vi "main_control_combo.vi"(6 "read":bool=TRUE) -> (9 "read string":string, 10 "bytes read":u32)   [LabVIEW 2019]
doc: "The Basic Serial Read and Write example performs a Serial Port Read, a Serial Port Write, or a combination of these actions. The user selects the actions (read or write) on the front panel. If both are selected, the VI will write the data first, read data, and then close the VISA session that is opened to the port. This VI will wait until the specified number of bytes is received at the port. Only the number of bytes specified will be read.\n\nINSTRUCTIONS:\n1) Select the serial resource and configuration parameters (baud rate, data bits, parity, stop bits, flow control).\n2) Select the operations to be performed. \n3) Connect the serial port to your device. If no device is available, perform a loopback test by doing one of the following. Short pins 2 and 3 on a RS-232 cable or short pin 4 to pin 8 and pin 5 to pin 9 on a RS-485/422 cable. \n4) Run the VI to see the data read. (The \"read string\" will match the \"string to write\" if a loopback test was performed.)\n\nNote: The parameters set for the serial port must match the parameters of the connected instrument or device. In this example, the bytes to read parameter specifies the number of bytes that the serial port reads. If there were more bytes at the port than the number specified in bytes to read, those bytes would not be read. Also, if you specify to read more bytes than the number of bytes actually read, you might receive a timeout error message.\n\nOn the block diagram, the Configure Serial Port VI sets the configuration parameters. The front panel displays the controls used to configure the basic parameters, such as baud rate, data bits, and parity. Constants configure the other parameters the user probably does not need set. After the VISA Configure Serial Port VI opens the VISA session and configures the port, the VI passes the VISA resource name to other VIs that perform operations on that VISA resource. The VISA Write function sends a command to the serial device and the VISA Read function returns data based on the command. The VISA Close function then closes the reference to the serial device. It is important to close the reference; otherwise communication through with that port through protocols other than VISA might not be possible."
uses:
  <vilib>/Instr/_visa.llb/VISA Configure Serial Port (Instr).vi
  <vilib>/Utility/file.llb/Read Delimited Spreadsheet (string).vi
  Keithley/Keithley 24XX/Public/Data/Read (Single Point).vi
  Keithley/Keithley 24XX/Keithley 24XX.lvlib
  DELTA ELEKTRONIKA SM Series/DELTA ELEKTRONIKA.lvlib
panel:
  out "Current Limit 2":bool
  out "Voltage Limit 2":bool
  out "bytes read 5":u32
  out "read string 5":string
  out "bytes read 4":u32
  out "read string 4":string
  out "standard output":string
  in  "Voltage Manual Range (1.0) 2":dbl=1.0
  in  "Current Manual Range (1.0) 2":dbl=1.0
  in  "Resistance Manual Range (1.0) 2":dbl=1.0
  in  "Enable Voltage Auto Range (T:Enable) 2":bool=TRUE
  in  "Enable Current Auto Range (T:Enable) 2":bool=TRUE
  in  "Enable Resistance Auto Range (T:Enable) 2":bool=TRUE
  out "Voltage 3":sgl
  out "Current 3":sgl
  out "Resistance 2":sgl
  out "Current Micro\n 2":sgl
  out "Command Log and Output":string
  out "COMBO COMMAND":string
  in  "Current Limit (0A)":dbl format="%.2f"
  in  "Voltage Level (0.0 V)":dbl format="%.2f"
  out "Actual Voltage Level (V)":dbl format="%.2f"
  out "Actual Current Limit (A)":dbl format="%.2f"
  out "Voltage Limit":bool
  out "Current Limit":bool
  out "all rows":string[][](array[string])
  out "element":i32
  out "subarray 4":string[](array[string])
  out "subarray 5":string[](array[string])
  out "size(s)":i32
  in  "file path (dialog if empty) 2":path
  in  "Read Script":bool
  in  "Voltage Manual Range (1.0)":dbl=1.0
  in  "Current Manual Range (1.0)":dbl=1.0
  in  "Resistance Manual Range (1.0)":dbl=1.0
  in  "Enable Voltage Auto Range (T:Enable)":bool=TRUE
  in  "Enable Current Auto Range (T:Enable)":bool=TRUE
  in  "Enable Resistance Auto Range (T:Enable)":bool=TRUE
  out "relay TTi":errorcluster
  out "bytes read 3":u32
  out "read string 3":string
  in  "read 3":bool=TRUE
  in  "delay before read (ms) 3":u32=500
  in  "Combo Box 3":string(combo)
  in  "voltage or current 2":dbl
  out "string from combo 3":string
  in  "write 3":bool
  out "LV TTi":errorcluster
  out "bytes read 2":u32
  out "read string 2":string
  in  "read 2":bool=TRUE
  in  "delay before read (ms) 2":u32=500
  in  "Combo Box 2":string(combo)="VO?\n"
  in  "voltage or current":dbl
  out "string from combo 2":string
  in  "write 2":bool
  in  "write":bool
  out "string from combo":string
  in  "Temperature":dbl
  in  "Combo Box":string(combo)
  out "Chiller":errorcluster
  out "N2 temperature > dew point + 2C":bool
  in  "File Path of rotonic datalog":path
  out "time humidity temporature dewpoint":string[](array[string])
  in  "Quit":bool
  in  "delay before read (ms)":u32=500
  # "Medical Chiller Interface\nCOM 6 is default"
  # "TTi LV powersupply Interface\nCOM 5 is default"
  # "TTi LV powersupply Interface for the relay polarity control\nCOM 4 is default"
  # "µA"
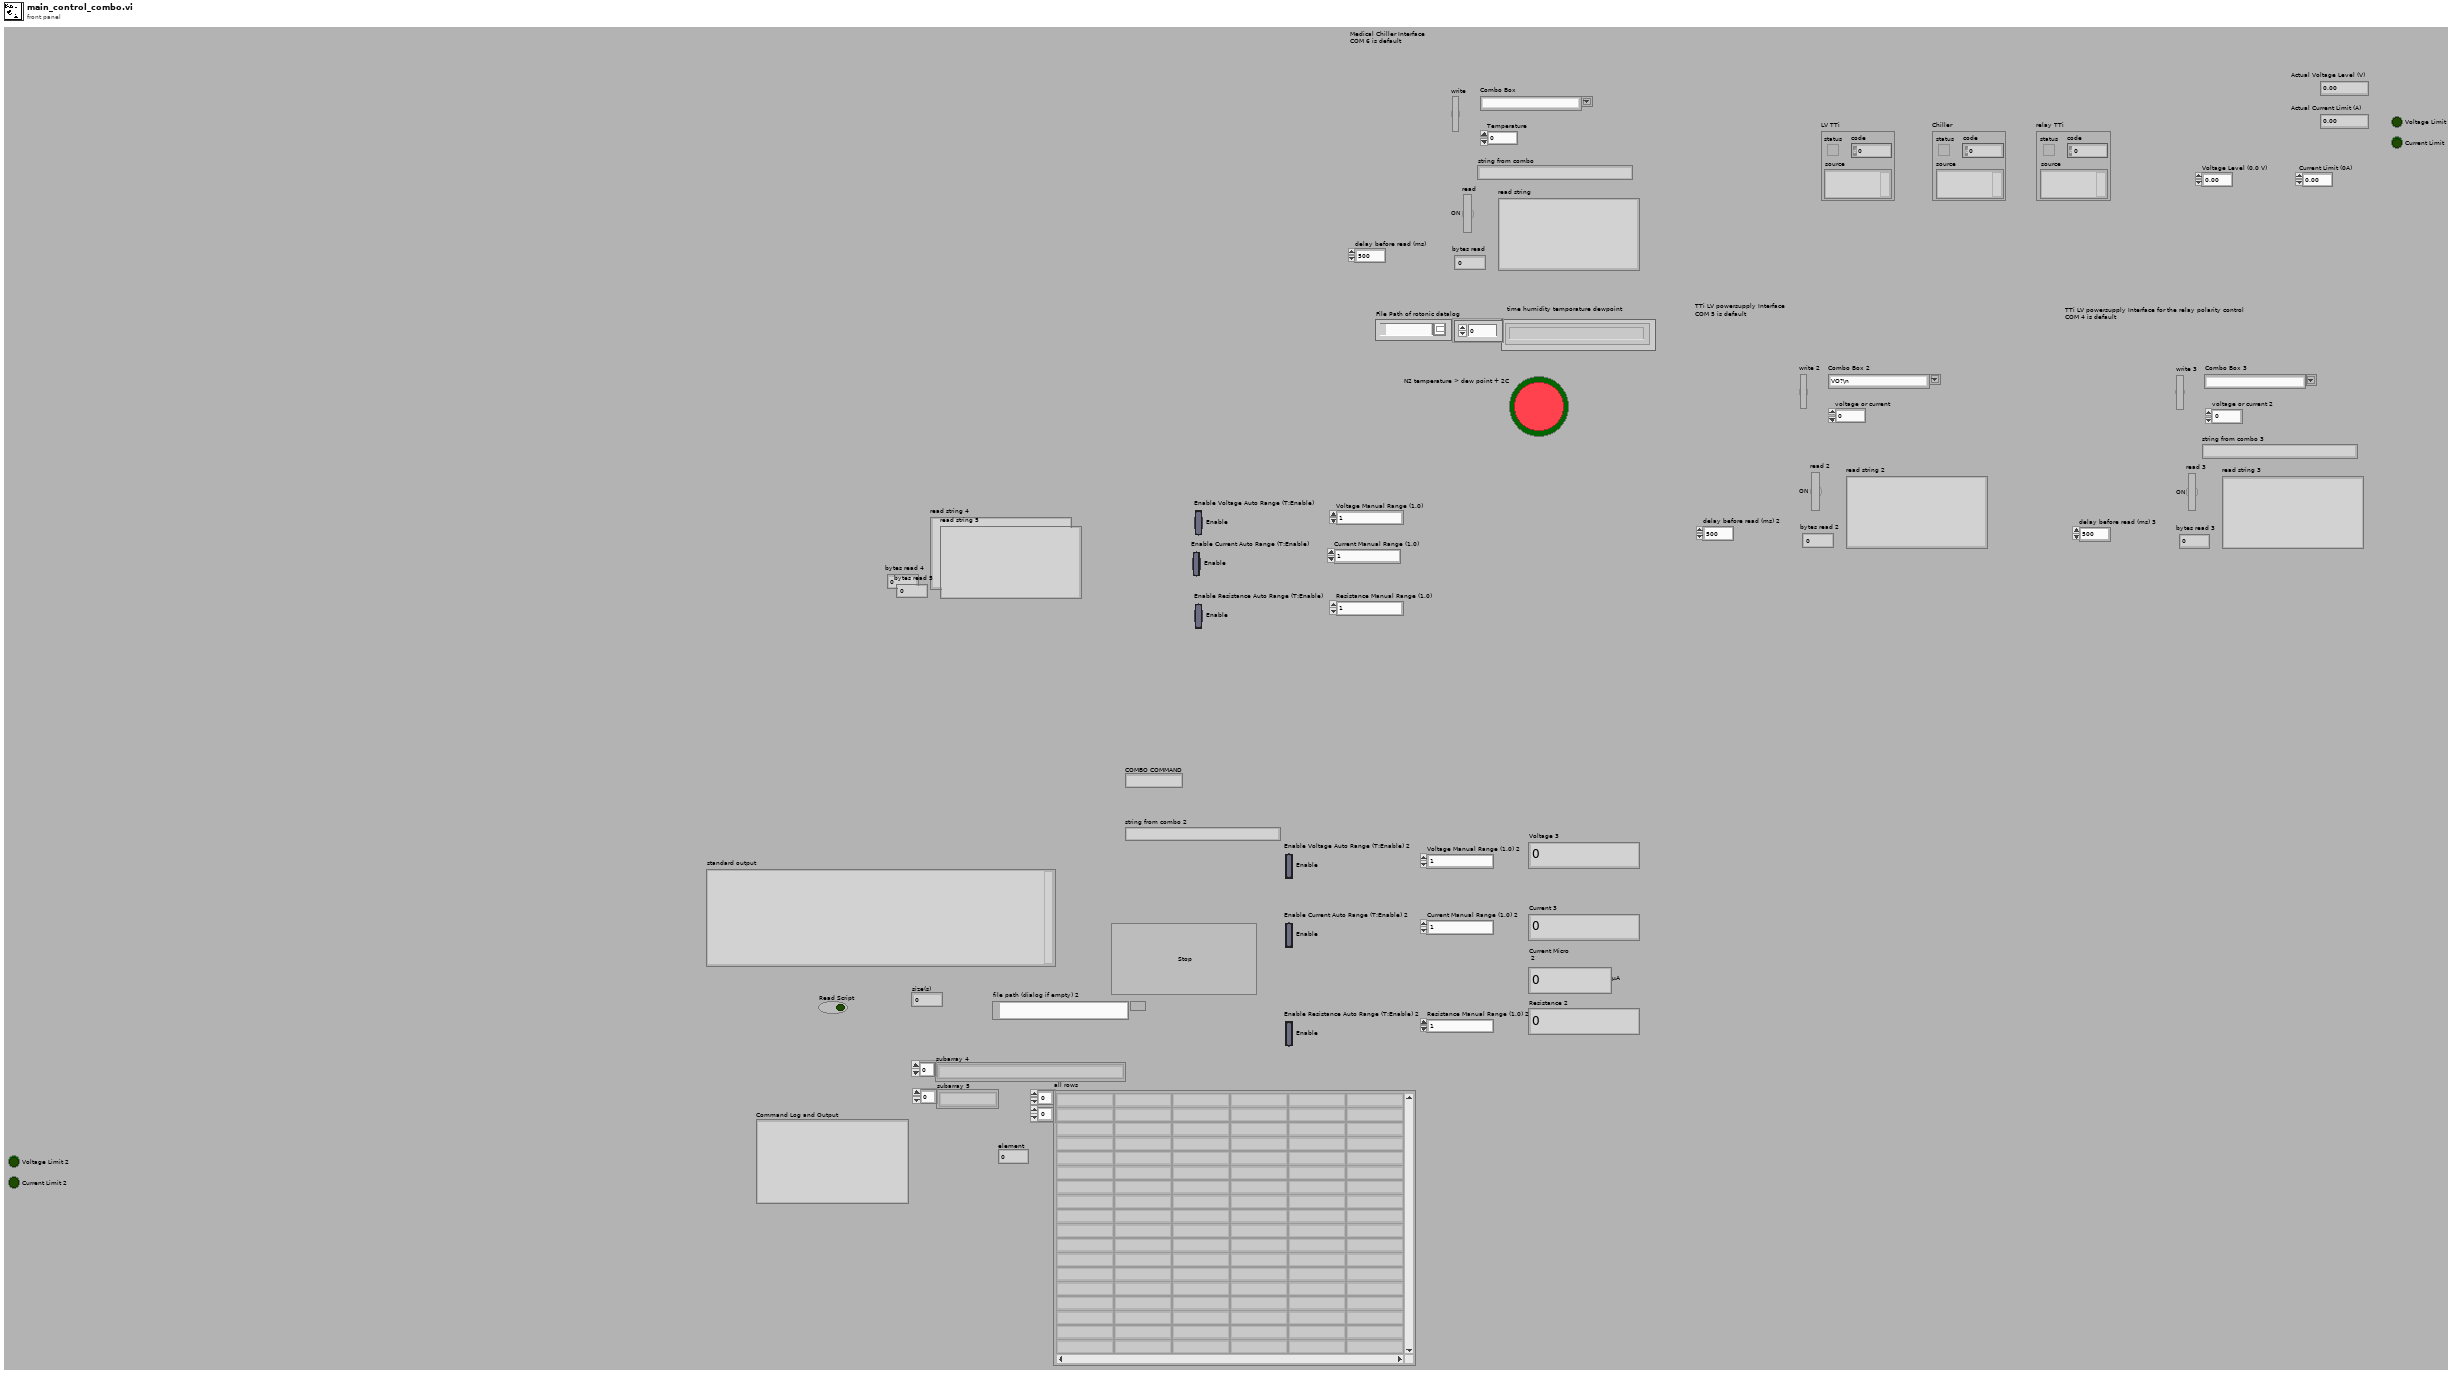
[diagram p1: front panel]
types:
  T1 = cluster{"Baud Rate":u32, "Parity":u16, "Data Bits":u16, "Stop Bits":u16, "Flow Control":u16}
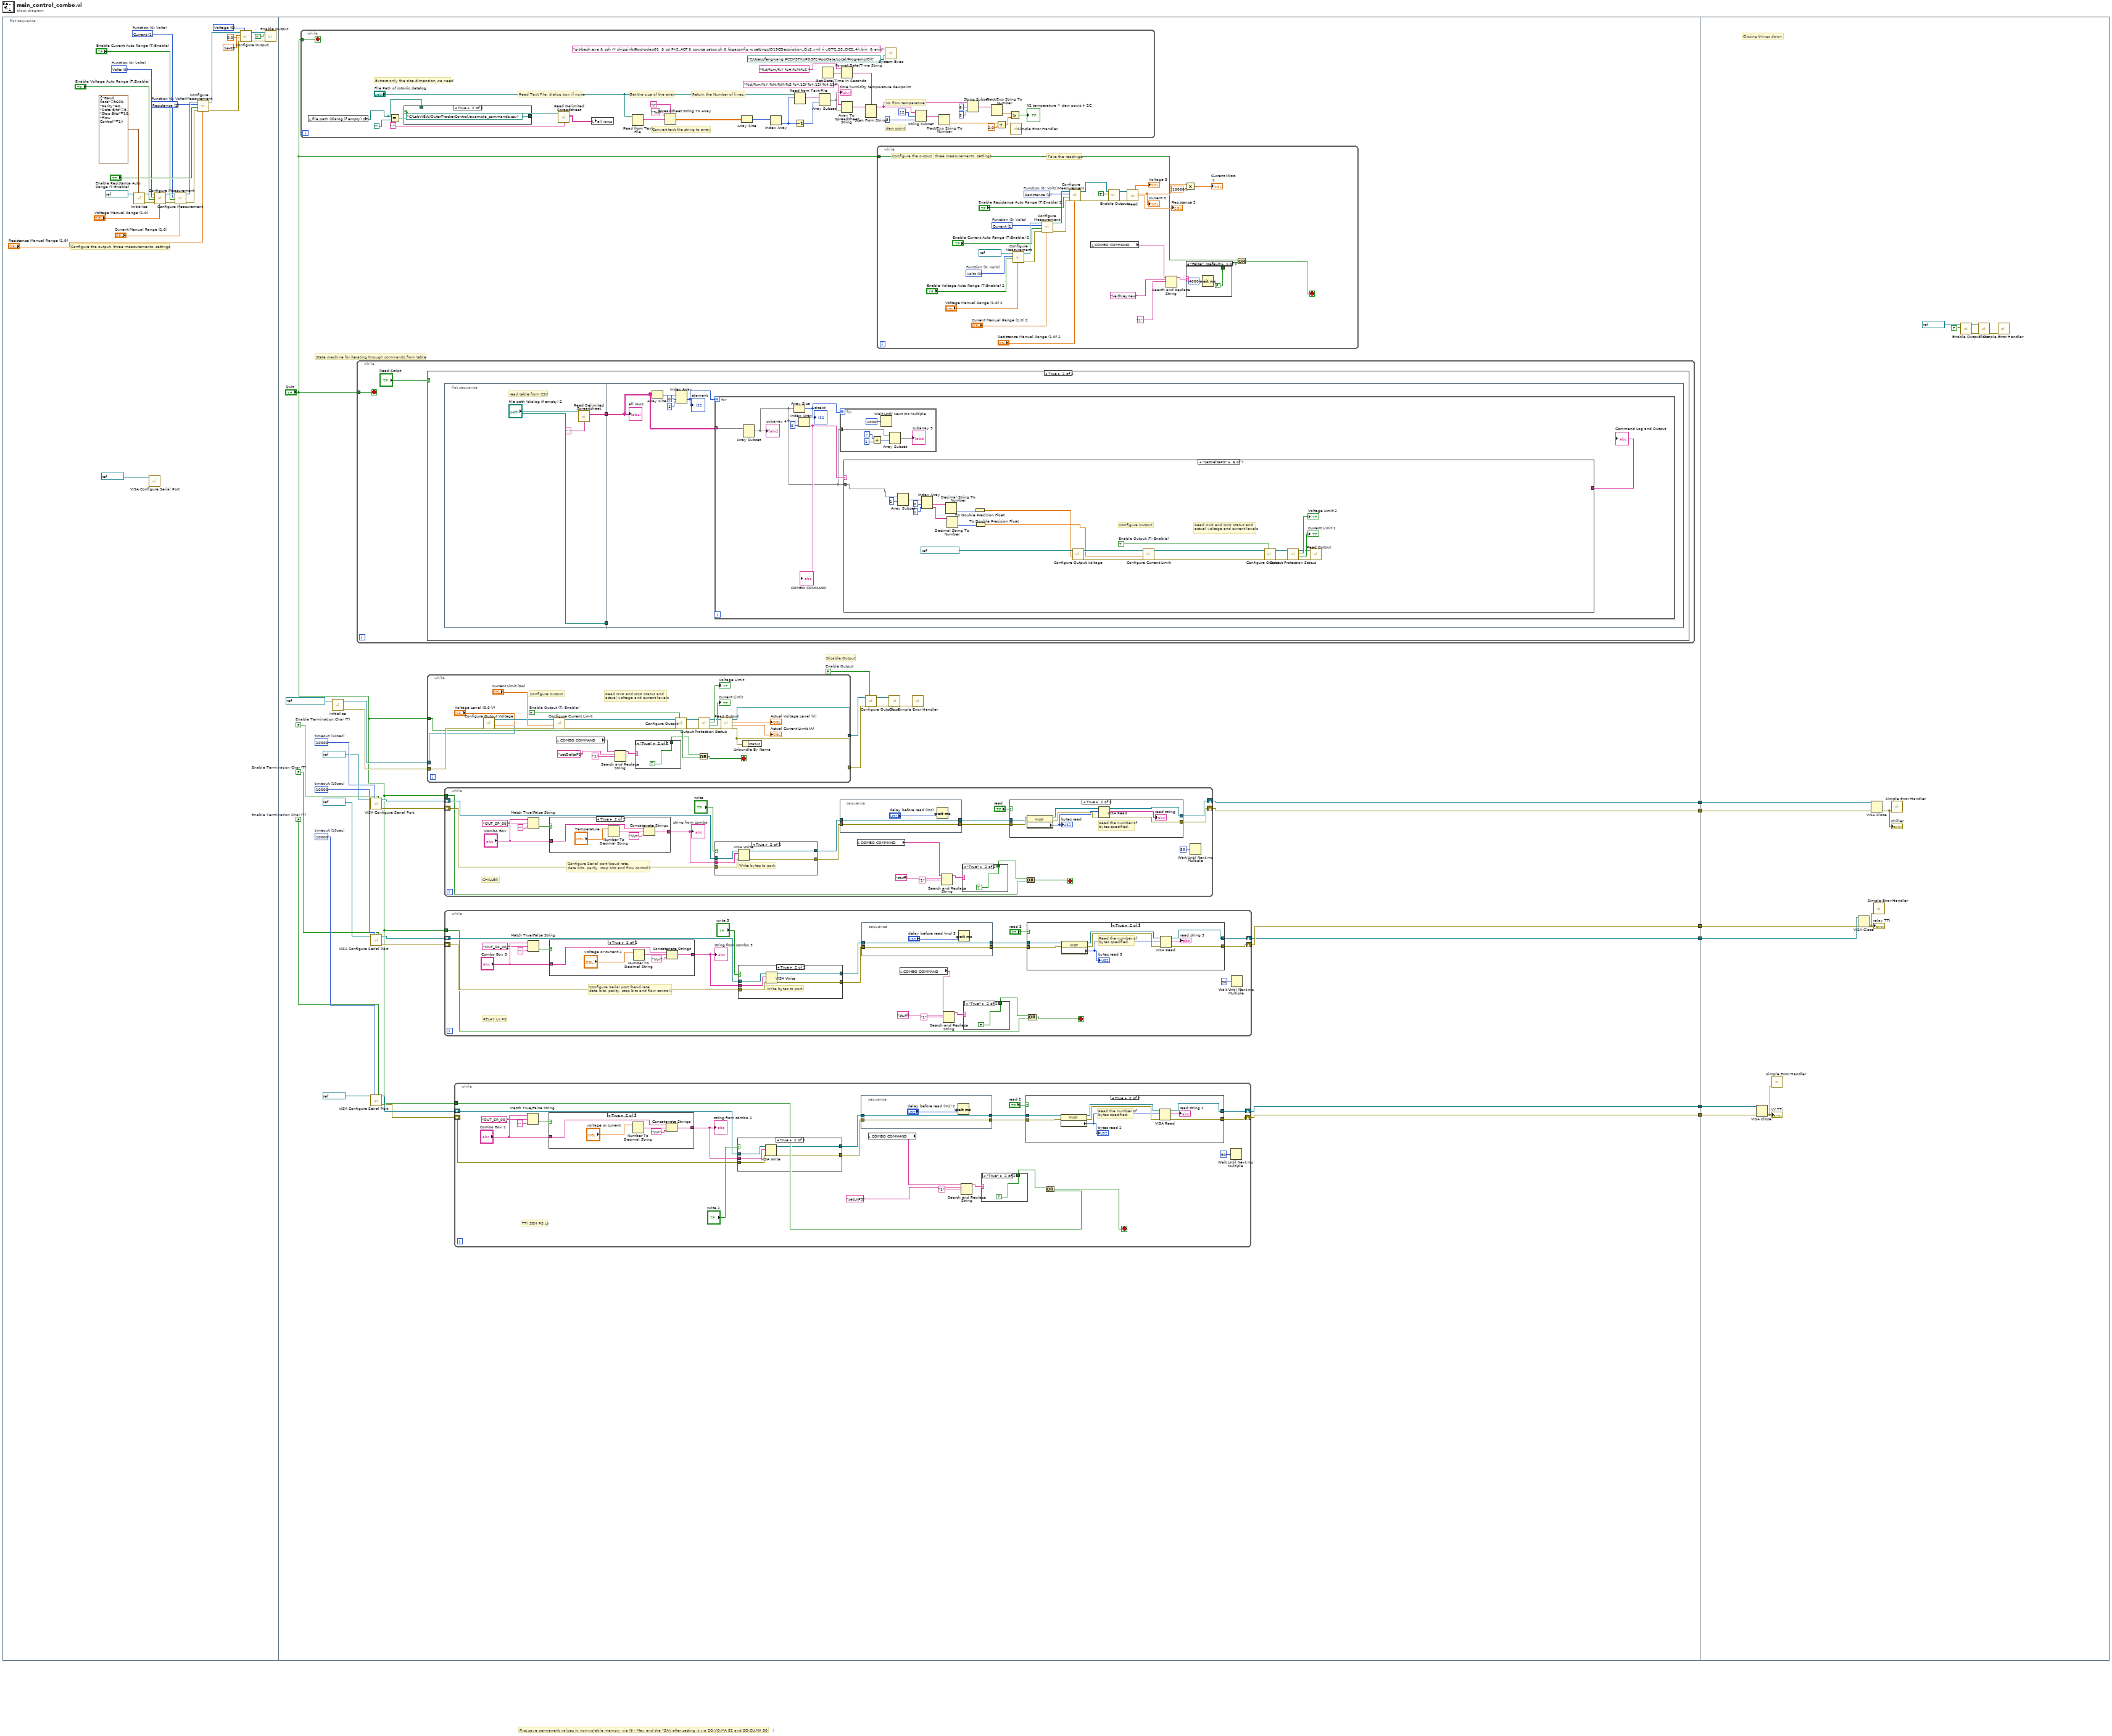
[diagram p0: block diagram]
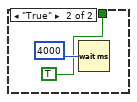
[diagram p2: hidden frame]
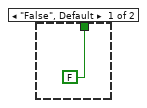
[diagram p3: hidden frame]
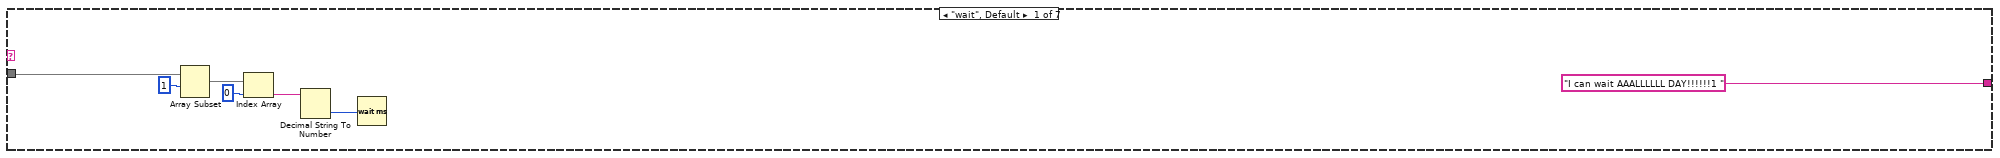
[diagram p5: hidden frame]
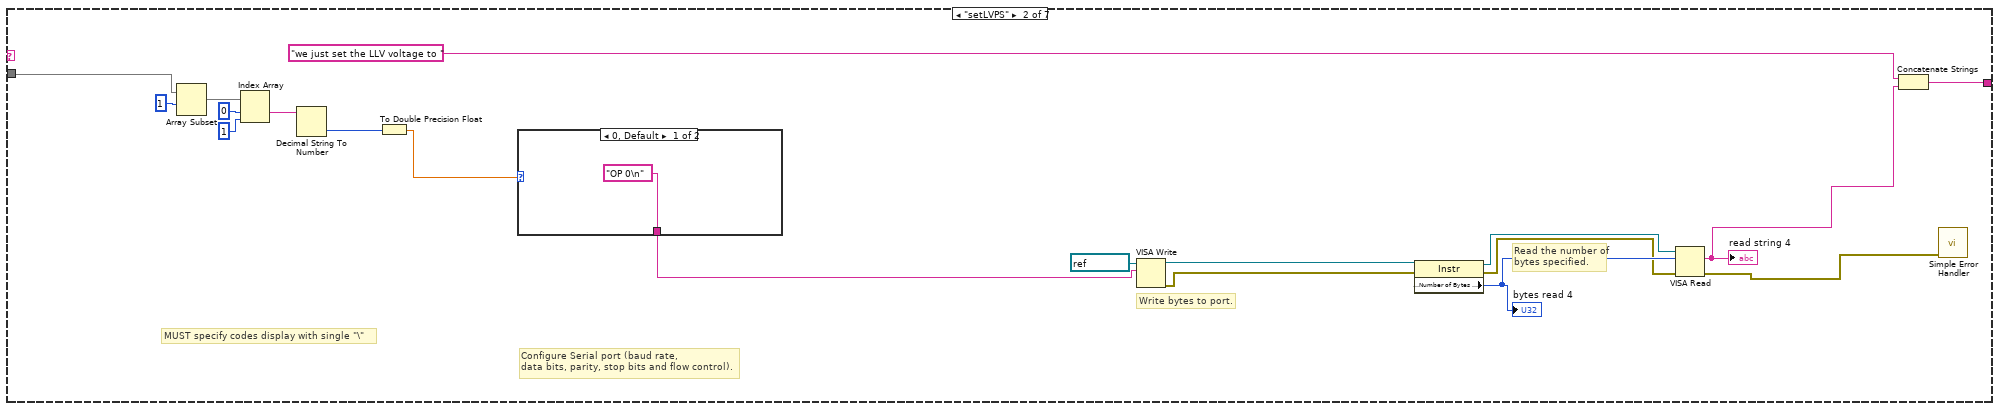
[diagram p6: hidden frame]
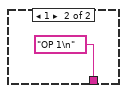
[diagram p7: hidden frame]
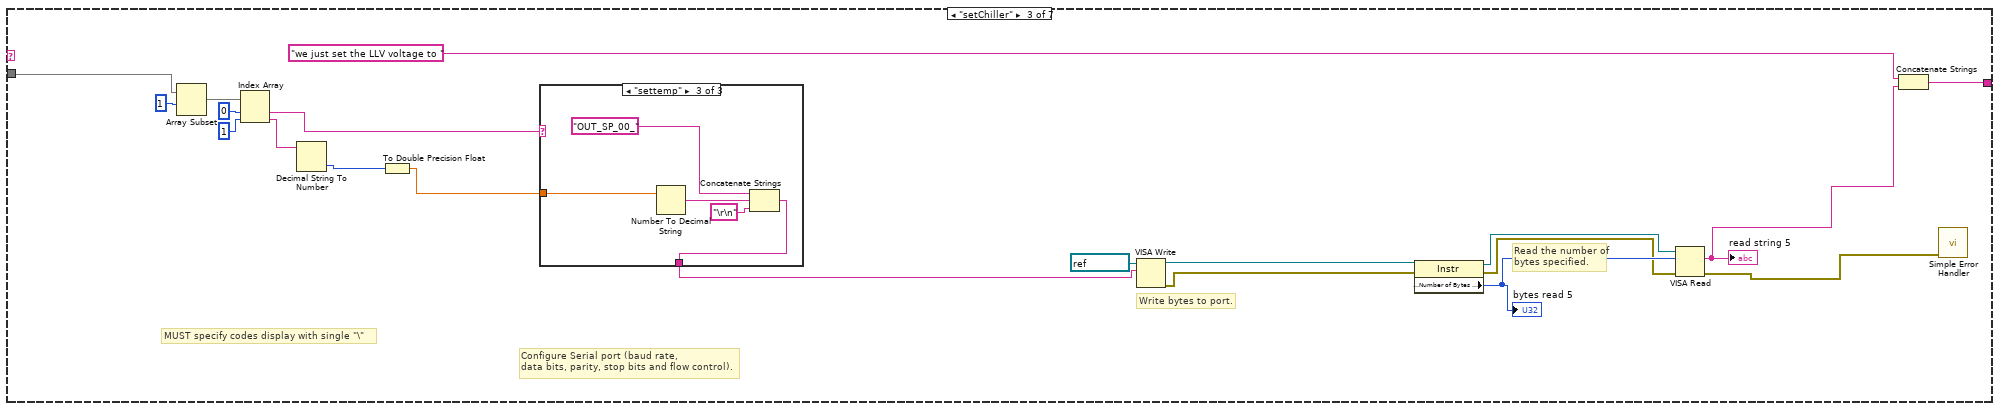
[diagram p8: hidden frame]
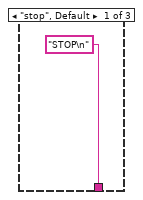
[diagram p9: hidden frame]
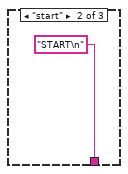
[diagram p10: hidden frame]
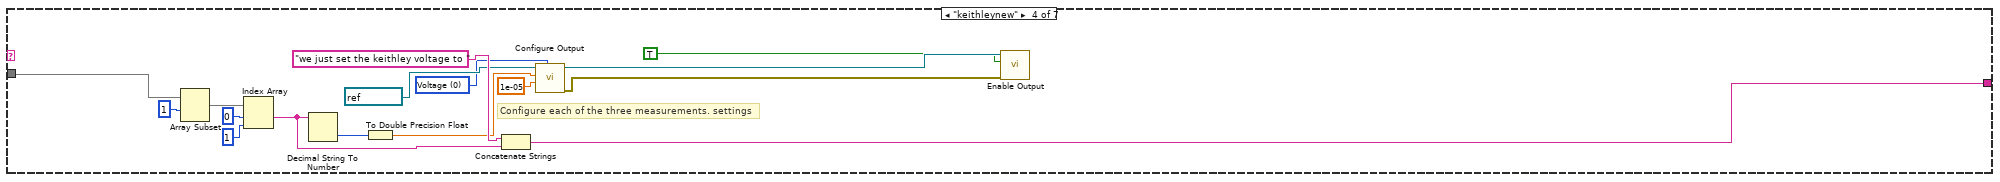
[diagram p11: hidden frame]
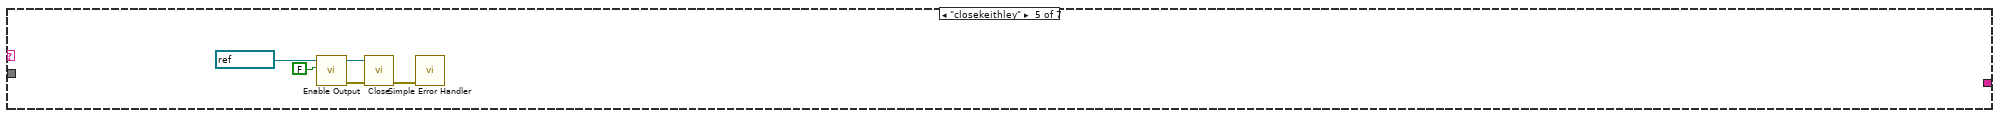
[diagram p12: hidden frame]
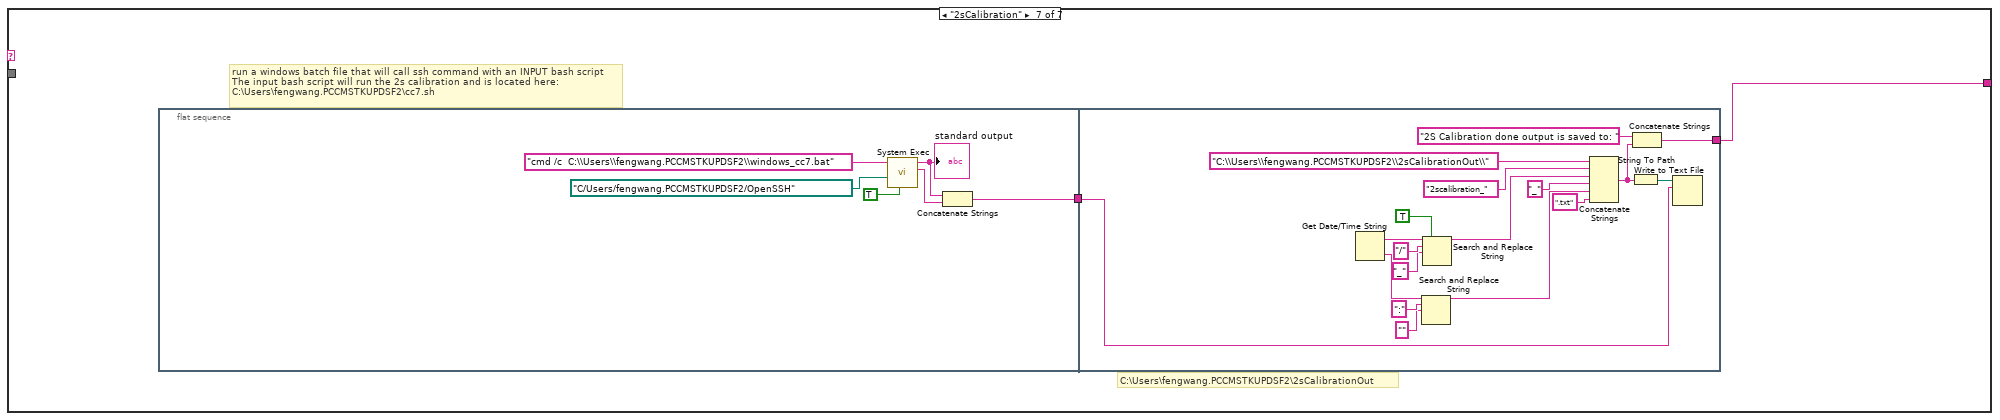
[diagram p13: hidden frame]
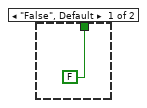
[diagram p14: hidden frame]
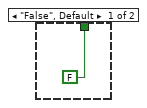
[diagram p18: hidden frame]
diagram:
  # "First save permanent values in non-volatile memory via NI - Max and the *SAV after setting it via SO:VO:MA 52 and SO:CU:MA 30    !"
  n1 = flat-sequence {
    tunnel: [w38] -> w6
    tunnel: [w37] -> w5
    tunnel: [w36] -> w4
    tunnel: [w35] -> w3
    tunnel: [w34] -> w2
    tunnel: [w33] -> w1
    tunnel: w6 -> [w474]
    tunnel: w5 -> [w473]
    tunnel: w4 -> [w471]
    tunnel: w3 -> [w470]
    tunnel: w2 -> [w468]
    tunnel: w1 -> [w467]
    frame #0 {
      w16 = u16 0 items=["Voltage", "Current"] ("Source Mode  (0: Voltage)")
      w9 = u16 0 items=["Volts", "Current", "Resistance"]  # Function (0: Volts)
      w12 = u16 2 items=["Volts", "Current", "Resistance"]  # Function (0: Volts)
      w11 = u16 1 items=["Volts", "Current", "Resistance"]  # Function (0: Volts)
      # "Configure the output."
      # "Configure each of the three measurements. settings"
      n2 = call "Initialize.vi"("Serial Configuration"=T1 {"Baud Rate"=9600, "Parity"=0, "Data Bits"=8, "Stop Bits"=10, "Flow Control"=1}, "VISA resource name"=refnum<visa-resource-name> "COM1" ("VISA resource name 4")) -> ("error out"=w10:errorcluster, "VISA resource name out"=w8:refnum<visa-resource-name>)  [unwired: 8 in]
      n3 = call-poly "VISA Configure Serial Port"("VISA resource name"=refnum<visa-resource-name> "COM5") -> ()  [unwired: 13 in, 2 out]
      n4 = call "Configure Measurement.vi"("Manual Range (1.0)"="Voltage Manual Range (1.0)", "error in (no error)"=w10, "Enable Auto Range (T:Enable)"="Enable Voltage Auto Range (T:Enable)", "Function (0: Volts)"=w9, "VISA resource name"=w8) -> ("error out"=w18:errorcluster, "VISA resource name out"=w17:refnum<visa-resource-name>)  [unwired: 5 in]
      n5 = call "Configure Measurement.vi"("Manual Range (1.0)"="Current Manual Range (1.0)", "error in (no error)"=w18, "Enable Auto Range (T:Enable)"="Enable Current Auto Range (T:Enable)", "Function (0: Volts)"=w11, "VISA resource name"=w17) -> ("error out"=w19:errorcluster, "VISA resource name out"=w20:refnum<visa-resource-name>)  [unwired: 5 in]
      n6 = call "Configure Measurement.vi"("Manual Range (1.0)"="Resistance Manual Range (1.0)", "error in (no error)"=w19, "Enable Auto Range (T:Enable)"="Enable Resistance Auto Range (T:Enable)", "Function (0: Volts)"=w12, "VISA resource name"=w20) -> ("error out"=w28:errorcluster, "VISA resource name out"=w27:refnum<visa-resource-name>)  [unwired: 5 in]
      n7 = call "Configure Output.vi"("Source Mode  (0: Voltage)"=w16, "error in (no error)"=w28, "Compliance  Level (0.1)"=1e-05, "Output Level (0)"=0.0, "VISA resource name"=w27) -> ("error out"=w29:errorcluster, "VISA resource name out"=w30:refnum<visa-resource-name>)  [unwired: 5 in]
      n8 = call "Enable Output.vi"("error in (no error)"=w29, "Enable Output (T: Enable)"=TRUE, "VISA resource name"=w30) -> ()  [unwired: 7 in, 2 out]
    }
    frame #1 {
      w46 = FALSE  # Enable Output
      w53 = FALSE  # Enable Termination Char (T)
      w54 = u32 10000  # timeout (10sec)
      w57 = FALSE  # Enable Termination Char (T)
      w58 = u32 10000  # timeout (10sec)
      w61 = FALSE  # Enable Termination Char (T)
      w62 = u32 10000  # timeout (10sec)
      # "Disable Output"
      # "State machine for iterating through commands from table"
      n9 = while {
        tunnel: "Quit" -> [w384]
        stop <- w384 stop-if-true
        # "dew point"
        # "N2 flow temperature"
        # "Convert text file string to array"
        # "Return the Number of lines."
        # "Extract only the size dimension we need"
        # "Get the size of the array"
        # "Read Text File, dialog box if none"
        n10 = local read "file path (dialog if empty) 2"() -> (w379:path)
        n11 = Equal?(x=w379, y=path "") -> (x = y?=w380:bool)
        n12 = case shown="True" w380 {
          tunnel: [w414 path "C:/LabVIEW/OuterTrackerControl/example_commands.csv"] -> w378
          tunnel: w379 -> [w414 _]
          frame False {
          }
          frame True {
          }
        }
        n13 = call-poly <vilib>:"Read Delimited Spreadsheet.vi"("file path (dialog if empty)"=w378, "delimiter (\\t)"="," ("delimiter (\\t)")) -> ("all rows"=w382:string[][])  [unwired: 8 in, 5 out]
        n14 = local write "all rows"(w382) -> ()
        n15 = Read from Text File(file (use dialog)="File Path of rotonic datalog") -> (text=w402:string)  [unwired: 1 in, 5 out]
        n16 = Spreadsheet String To Array(delimiter (Tab)="\r", format string="%d", spreadsheet string=w402) -> (array=w400:dbl[][])  [unwired: 1 out]
        n17 = Array Size(array=w400) -> (size(s)=w401:i32[])
        n18 = Index Array(array=w401) -> (element=w405:i32)  [unwired: 1 in]
        n19 = Read from Text File(file (use dialog)="File Path of rotonic datalog", count=w405) -> (text=w406:string[])  [unwired: 1 in, 4 out]
        n20 = Decrement(x=w405) -> (x-1=w403:i32)
        n21 = Array Subset(array=w406, index=w403) -> (w407:string[])  [unwired: 1 in]
        "time humidity temporature dewpoint" <- w407
        n22 = Get Date/Time In Seconds() -> (seconds since 1Jan1904=w398:timestamp)
        n23 = Format Date/Time String(time format string (%c)="%d/%m/%Y %H:%M:%S ", seconds (now)=w398) -> (date/time string=w399:string)  [unwired: 1 in]
        n24 = Array To Spreadsheet String(array=w407, 3:"%d/%m/%Y %H:%M:%S %4.12f %4.12f %4.12f" ("time format string (%c)")) -> (spreadsheet string=w408:string)  [unwired: 1 in]
        n25 = Scan From String(format string=w399, input string=w408) -> (remaining string=w409:string)  [unwired: 4 in, 2 out]
        n26 = call <vilib>:"System Exec.vi"("working directory"=path "C:/Users/fengwang.PCCMSTKUPDSF2/AppData/Local/Programs/Git", "command line"="git-bash.exe & ssh -Y shigginb@pchpdaq01  & cd Ph2_ACF & source setup.sh & fpgaconfig -c settings/D19CDescription_Cic2.xml -i uDTC_2S_CIC2_4h.bin  & exit") -> ()  [unwired: 6 in, 4 out]
        n27 = String Subset(string=w409, offset (0)=12, length (rest)=5 ("length (rest)")) -> (substring=w411:string)
        n28 = Fract/Exp String To Number(string=w411) -> (number=w388:dbl)  [unwired: 3 in, 1 out]
        n29 = String Subset(string=w409, offset (0)=6, length (rest)=5 ("length (rest)")) -> (substring=w410:string)
        n30 = Fract/Exp String To Number(string=w410) -> (number=w412:dbl)  [unwired: 3 in, 1 out]
        n31 = Add(x=w388, y=2.0) -> (x+y=w387:dbl)
        n32 = Greater?(x=w412, y=w387) -> (0:→"N2 temperature > dew point + 2C":bool)
        n33 = call <vilib>:"Simple Error Handler.vi"() -> ()  [unwired: 5 in, 5 out]
      }
      n34 = call "Initialize.vi"("VISA resource name"=refnum<visa-resource-name> "GPIB0::8::INSTR") -> ("error out"=w51:errorcluster, "VISA resource name out"=w50:refnum<visa-resource-name>)  [unwired: 9 in]
      n35 = while {
        tunnel: "Quit" -> [w127]
        stop <- w127 stop-if-true
        n36 = case shown="True" "Read Script" {
          frame False {
          }
          frame True {
            n37 = flat-sequence {
              tunnel: ["file path (dialog if empty) 2"] -> w130
              tunnel: [w132] -> w129
              tunnel: w130 -> [_]
              tunnel: w129 -> [w134]
              frame #0 {
                # "read table from CSV"
                n38 = call-poly <vilib>:"Read Delimited Spreadsheet.vi"("file path (dialog if empty)"="file path (dialog if empty) 2", "delimiter (\\t)"="," ("delimiter (\\t)")) -> ("all rows"=w132:string[][])  [unwired: 8 in, 5 out]
              }
              frame #1 {
                n39 = Array Size(array=w134) -> (size(s)=w137:i32[])
                n40 = Index Array(array=w137, index #1=0 ("index"), index #2=1 ("index")) -> (element #1=w138:i32)  [unwired: 1 out]
                "element" <- w138
                n41 = for {
                  N: w138 -> [_]
                  tunnel: w134 -> [w144] mode=indexing
                  n42 = Array Subset(array=w144) -> (w140:string[])  [unwired: 2 in]
                  "subarray 4" <- w140
                  n43 = Array Size(array=w140) -> (size(s)=w143:i32)
                  "size(s)" <- w143
                  n44 = Index Array(array=w140, index=0) -> (element=w141:string)
                  "COMBO COMMAND" <- w141
                  n45 = for {
                    N: w143 -> [_]
                    tunnel: w140 -> [w274]
                    i -> [w271]
                    n46 = Add(x=w271, y=1) -> (x+y=w270:i32)
                    n47 = Wait Until Next ms Multiple(millisecond multiple=u32 1000) -> ()  [unwired: 1 out]
                    n48 = Array Subset(array=w274, index=w270) -> (→"subarray 5":string[])  [unwired: 1 in]
                  }
                  n49 = case shown="\"setDeltaPS\"" w141 {
                    tunnel: w140 -> [w151 w165 w188 w212 _ w226 _]
                    tunnel: ["I can wait AAALLLLLL DAY!!!!!!1 " w162 w186 w208 _ _ w244] -> w139
                    frame "wait", Default {
                      n50 = Array Subset(array=w151, index=1) -> (w149:string[])  [unwired: 1 in]
                      n51 = Index Array(array=w149, index=0) -> (element=w147:string)
                      n52 = Decimal String To Number(string=w147) -> (number=w146:i32)  [unwired: 2 in, 1 out]
                      n53 = Wait (ms)(milliseconds to wait=w146) -> ()  [unwired: 1 out]
                    }
                    frame "setLVPS" {
                      # "Read the number of bytes specified."
                      # "Write bytes to port."
                      # "MUST specify codes display with single \"\\\""
                      # "Configure Serial port (baud rate,\ndata bits, parity, stop bits and flow control)."
                      n54 = Array Subset(array=w165, index=1) -> (w170:string[])  [unwired: 1 in]
                      n55 = Index Array(array=w170, index #1=0 ("index"), index #2=1 ("index")) -> (element #1=w167:string)  [unwired: 1 out]
                      n56 = Decimal String To Number(string=w167) -> (number=w164:i32)  [unwired: 2 in, 1 out]
                      n57 = To Double Precision Float(number=w164) -> (double precision float=w161:dbl)
                      n58 = case shown="0, Default" w161 {
                        tunnel: ["OP 0\n" ("Combo Box 4") "OP 1\n" ("Combo Box 4")] -> w160
                        frame 0, Default {
                        }
                        frame 1 {
                        }
                      }
                      n59 = VISA Write(VISA resource name=refnum<visa-resource-name> "COM5", write buffer=w160) -> (VISA resource name out=w153:refnum<visa-resource-name>, error out=w152:errorcluster)  [unwired: 1 in, 1 out]
                      n60 = property class="Instr"(reference=w153, error in=w152) -> (reference out=w155:refnum<visa-resource-name>, error out=w156:errorcluster, "Serial Settings:Number of Bytes at Serial Port"=w157:u32)
                      "bytes read 4" <- w157
                      n61 = VISA Read(VISA resource name=w155, byte count=w157, error in (no error)=w156) -> (read buffer=w158:string, error out=w154:errorcluster)  [unwired: 2 out]
                      "read string 4" <- w158
                      n62 = Concatenate Strings("we just set the LLV voltage to ", w158) -> (w162:string)
                      n63 = call <vilib>:"Simple Error Handler.vi"("error in (no error)"=w154) -> ()  [unwired: 4 in, 5 out]
                    }
                    frame "setChiller" {
                      # "Read the number of bytes specified."
                      # "Write bytes to port."
                      # "MUST specify codes display with single \"\\\""
                      # "Configure Serial port (baud rate,\ndata bits, parity, stop bits and flow control)."
                      n64 = Array Subset(array=w188, index=1) -> (w192:string[])  [unwired: 1 in]
                      n65 = Index Array(array=w192, index #1=0 ("index"), index #2=1 ("index")) -> (element #1=w174:string, element #2=w176:string)
                      n66 = Decimal String To Number(string=w176) -> (number=w175:i32)  [unwired: 2 in, 1 out]
                      n67 = To Double Precision Float(number=w175) -> (double precision float=w173:dbl)
                      n68 = case shown="\"settemp\"" w174 {
                        tunnel: ["STOP\n" ("Combo Box 4") "START\n" ("Combo Box 4") w196] -> w185
                        tunnel: w173 -> [_ _ w195]
                        frame "stop", Default {
                        }
                        frame "start" {
                        }
                        frame "settemp" {
                          n69 = Number To Decimal String(number=w195) -> (decimal integer string=w199:string)  [unwired: 1 in]
                          n70 = Concatenate Strings("OUT_SP_00_" ("Combo Box 4"), w199, "\r\n" ("string")) -> (w196:string)
                        }
                      }
                      n71 = VISA Write(VISA resource name=refnum<visa-resource-name> "COM6", write buffer=w185) -> (VISA resource name out=w178:refnum<visa-resource-name>, error out=w177:errorcluster)  [unwired: 1 in, 1 out]
                      n72 = property class="Instr"(reference=w178, error in=w177) -> (reference out=w180:refnum<visa-resource-name>, error out=w181:errorcluster, "Serial Settings:Number of Bytes at Serial Port"=w182:u32)
                      "bytes read 5" <- w182
                      n73 = VISA Read(VISA resource name=w180, byte count=w182, error in (no error)=w181) -> (read buffer=w183:string, error out=w179:errorcluster)  [unwired: 2 out]
                      "read string 5" <- w183
                      n74 = Concatenate Strings("we just set the LLV voltage to ", w183) -> (w186:string)
                      n75 = call <vilib>:"Simple Error Handler.vi"("error in (no error)"=w179) -> ()  [unwired: 4 in, 5 out]
                    }
                    frame "keithleynew" {
                      w200 = u16 0 items=["Voltage", "Current"] ("Source Mode  (0: Voltage)")
                      # "Configure each of the three measurements. settings"
                      n76 = Array Subset(array=w212, index=1) -> (w215:string[])  [unwired: 1 in]
                      n77 = Index Array(array=w215, index #1=0 ("index"), index #2=1 ("index")) -> (element #1=w209:string)  [unwired: 1 out]
                      n78 = Decimal String To Number(string=w209) -> (number=w211:i32)  [unwired: 2 in, 1 out]
                      n79 = To Double Precision Float(number=w211) -> (double precision float=w206:dbl)
                      n80 = Concatenate Strings("we just set the keithley voltage to ", w209) -> (w208:string)
                      n81 = call "Configure Output.vi"("Source Mode  (0: Voltage)"=w200, "Compliance  Level (0.1)"=1e-05, "Output Level (0)"=w206, "VISA resource name"=refnum<visa-resource-name> "COM1") -> ("error out"=w204:errorcluster, "VISA resource name out"=w205:refnum<visa-resource-name>)  [unwired: 6 in]
                      n82 = call "Enable Output.vi"("error in (no error)"=w204, "Enable Output (T: Enable)"=TRUE, "VISA resource name"=w205) -> ()  [unwired: 7 in, 2 out]
                    }
                    frame "closekeithley" {
                      n83 = call "Enable Output.vi"("Enable Output (T: Enable)"=FALSE, "VISA resource name"=refnum<visa-resource-name> "COM1") -> ("error out"=w217:errorcluster, "VISA resource name out"=w218:refnum<visa-resource-name>)  [unwired: 8 in]
                      n84 = call "Close.vi"("error in (no error)"=w217, "VISA resource name"=w218) -> ("error out"=w220:errorcluster)  [unwired: 9 in]
                      n85 = call <vilib>:"Simple Error Handler.vi"("error in (no error)"=w220) -> ()  [unwired: 4 in, 5 out]
                    }
                    frame "setDeltaPS" {
                      w241 = TRUE  # Enable Output (T: Enable)
                      # "Read OVP and OCP Status and\nactual voltage and current levels"
                      # "Configure Output"
                      n86 = Array Subset(array=w226, index=1) -> (w231:string[])  [unwired: 1 in]
                      n87 = Index Array(array=w231, index #1=0 ("index"), index #2=1 ("index")) -> (element #1=w228:string, element #2=w223:string)
                      n88 = Decimal String To Number(string=w228) -> (number=w225:i32)  [unwired: 2 in, 1 out]
                      n89 = Decimal String To Number(string=w223) -> (number=w224:i32)  [unwired: 2 in, 1 out]
                      n90 = To Double Precision Float(number=w225) -> (double precision float=w221:dbl)
                      n91 = To Double Precision Float(number=w224) -> (double precision float=w222:dbl)
                      n92 = call "Configure Output Voltage.vi"("Set Voltage(0.0 V)"=w221, "VISA resource name"=refnum<visa-resource-name> "GPIB0::8::INSTR") -> ("error out"=w240:errorcluster, "VISA resource name out"=w239:refnum<visa-resource-name>)  [unwired: 8 in]
                      n93 = call "Configure Current Limit.vi"("error in (no error)"=w240, "Current Limit (0.0 A)"=w222, "VISA resource name"=w239) -> ("error out"=w242:errorcluster, "VISA resource name out"=w243:refnum<visa-resource-name>)  [unwired: 7 in]
                      n94 = call "Configure Output.vi"("Enable Output (T: Enable)"=w241, "error in (no error)"=w242, "VISA resource name"=w243) -> ("error out"=w233:errorcluster, "VISA resource name out"=w232:refnum<visa-resource-name>)  [unwired: 7 in]
                      n95 = call "Output Protection Status.vi"("error in (no error)"=w233, "VISA resource name"=w232) -> ("error out"=w235:errorcluster, "OCP Tripped?"=→"Current Limit 2":bool, "OVP Tripped?"=→"Voltage Limit 2":bool, "VISA resource name out"=w234:refnum<visa-resource-name>)  [unwired: 6 in]
                      n96 = call "Read Output.vi"("error in (no error)"=w235, "VISA resource name"=w234) -> ()  [unwired: 6 in, 4 out]
                    }
                    frame "2sCalibration" {
                      # "C:\\Users\\fengwang.PCCMSTKUPDSF2\\2sCalibrationOut"
                      # "run a windows batch file that will call ssh command with an INPUT bash script\nThe input bash script will run the 2s calibration and is located here:\nC:\\Users\\fengwang.PCCMSTKUPDSF2\\cc7.sh"
                      n97 = flat-sequence {
                        tunnel: [w247] -> w245
                        tunnel: w245 -> [w253]
                        tunnel: [w252] -> w244
                        frame #0 {
                          n98 = call <vilib>:"System Exec.vi"("run minimized? (F)"=TRUE, "working directory"=path "C:/Users/fengwang.PCCMSTKUPDSF2/OpenSSH", "command line"="cmd /c  C:\\Users\\fengwang.PCCMSTKUPDSF2\\windows_cc7.bat") -> ("standard error"=w248:string, "standard output"=w249:string)  [unwired: 5 in, 2 out]
                          "standard output" <- w249
                          n99 = Concatenate Strings(w249, w248) -> (w247:string)
                        }
                        frame #1 {
                          n100 = Get Date/Time String() -> (date string=w264:string, time string=w266:string)  [unwired: 3 in]
                          n101 = Search and Replace String(input string=w266, search string=":", replace string="" ("replace string (\"\")")) -> (result string=w267:string)  [unwired: 5 in, 3 out]
                          n102 = Search and Replace String(replace all?=TRUE ("replace all? (F)"), input string=w264, search string="/", replace string="_" ("replace string (\"\")")) -> (result string=w265:string)  [unwired: 4 in, 3 out]
                          n103 = Concatenate Strings("C:\\Users\\fengwang.PCCMSTKUPDSF2\\2sCalibrationOut\\" ("string"), "2scalibration_" ("string"), w265, "_" ("string"), w267, ".txt" ("string")) -> (w268:string)
                          n104 = String To Path(string=w268) -> (path=w269:path)
                          n105 = Concatenate Strings("2S Calibration done output is saved to: ", w268) -> (w252:string)
                          n106 = Write to Text File(file (use dialog)=w269, text=w253) -> ()  [unwired: 2 in, 3 out]
                        }
                      }
                    }
                  }
                  "Command Log and Output" <- w139
                }
                "all rows" <- w134
              }
            }
          }
        }
      }
      n107 = call-poly "VISA Configure Serial Port"("VISA resource name"=refnum<visa-resource-name> "COM6", "timeout (10sec)"=w62, "Enable Termination\nChar (T)"=w61) -> ("VISA resource name out"=w63:refnum<visa-resource-name>, "error out"=w60:errorcluster)  [unwired: 11 in]
      n108 = call-poly "VISA Configure Serial Port"("VISA resource name"=refnum<visa-resource-name> "COM4", "timeout (10sec)"=w54, "Enable Termination\nChar (T)"=w53) -> ("VISA resource name out"=w55:refnum<visa-resource-name>, "error out"=w52:errorcluster)  [unwired: 11 in]
      n109 = call-poly "VISA Configure Serial Port"("VISA resource name"=refnum<visa-resource-name> "COM5", "timeout (10sec)"=w58, "Enable Termination\nChar (T)"=w57) -> ("VISA resource name out"=w59:refnum<visa-resource-name>, "error out"=w56:errorcluster)  [unwired: 11 in]
      n110 = while {
        tunnel: w51 -> [w117]
        tunnel: w50 -> [w116]
        tunnel: [w107] -> w45
        tunnel: [w106] -> w44
        tunnel: "Quit" -> [w105]
        stop <- w99 stop-if-true
        w121 = TRUE  # Enable Output (T: Enable)
        # "Read OVP and OCP Status and\nactual voltage and current levels"
        # "Configure Output"
        n111 = call "Configure Output Voltage.vi"("error in (no error)"=w117, "Set Voltage(0.0 V)"="Voltage Level (0.0 V)", "VISA resource name"=w116) -> ("error out"=w120:errorcluster, "VISA resource name out"=w119:refnum<visa-resource-name>)  [unwired: 7 in]
        n112 = call "Configure Current Limit.vi"("error in (no error)"=w120, "Current Limit (0.0 A)"="Current Limit (0A)", "VISA resource name"=w119) -> ("error out"=w123:errorcluster, "VISA resource name out"=w124:refnum<visa-resource-name>)  [unwired: 7 in]
        n113 = local read "COMBO COMMAND"() -> (w100:string)
        n114 = Search and Replace String(input string=w100, search string="setDeltaPS", replace string="1" ("replace string (\"\")")) -> (result string=w103:string)  [unwired: 5 in, 3 out]
        n115 = case shown="\"True\"" w103 {
          tunnel: [FALSE TRUE] -> w104
          frame "False", Default {
          }
          frame "True" {
          }
        }
        n116 = call "Configure Output.vi"("Enable Output (T: Enable)"=w121, "error in (no error)"=w123, "VISA resource name"=w124) -> ("error out"=w109:errorcluster, "VISA resource name out"=w108:refnum<visa-resource-name>)  [unwired: 7 in]
        n117 = Or(x=w104, y=w105) -> (x .or. y?=w99:bool)
        n118 = call "Output Protection Status.vi"("error in (no error)"=w109, "VISA resource name"=w108) -> ("error out"=w111:errorcluster, "OCP Tripped?"=→"Current Limit":bool, "OVP Tripped?"=→"Voltage Limit":bool, "VISA resource name out"=w110:refnum<visa-resource-name>)  [unwired: 6 in]
        n119 = call "Read Output.vi"("error in (no error)"=w111, "VISA resource name"=w110) -> ("error out"=w106:errorcluster, "Actual Current Level (A)"=→"Actual Current Limit (A)":dbl, "Actual Voltage Level (V)"=→"Actual Voltage Level (V)":dbl, "VISA resource name out"=w107:refnum<visa-resource-name>)  [unwired: 6 in]
        n120 = Unbundle By Name(w106) -> ()  [unwired: 1 out]
      }
      n121 = while {
        shift-right: [w435] -> w38
        shift-left: w60 -> [w437]
        shift-right: [w434] -> w37
        shift-left: w63 -> [w436]
        tunnel: "Quit" -> [w418]
        stop <- w417 stop-if-true
        # "CHILLER"
        # "Configure Serial port (baud rate,\ndata bits, parity, stop bits and flow control)."
        n122 = Match True/False String(2:"" ("false string"), 3:"OUT_SP_00_" ("format string"), 4:"Combo Box") -> (0:w427:bool)  [unwired: 1 out]
        n123 = case shown="True" w427 {
          tunnel: [w441 w444] -> w424
          tunnel: "Combo Box" -> [w441 w443]
          frame False {
          }
          frame True {
            n124 = Number To Decimal String(number="Temperature") -> (decimal integer string=w446:string)  [unwired: 1 in]
            n125 = Concatenate Strings(w443, w446, "\r\n" ("string")) -> (w444:string)
          }
        }
        "string from combo" <- w424
        n126 = case shown="True" "write" {
          tunnel: [w451 w456] -> w433
          tunnel: w436 -> [w450 w455]
          tunnel: w437 -> [w451 w454]
          tunnel: [w450 w453] -> w431
          tunnel: w424 -> [_ w452]
          frame False {
          }
          frame True {
            # "Write bytes to port."
            n127 = VISA Write(VISA resource name=w455, write buffer=w452, error in (no error)=w454) -> (VISA resource name out=w453:refnum<visa-resource-name>, error out=w456:errorcluster)  [unwired: 1 out]
          }
        }
        n128 = stacked-sequence {
          tunnel: w433 -> [w449]
          tunnel: [w449] -> w432
          tunnel: w431 -> [w448]
          tunnel: [w448] -> w430
          frame #0 {
            n129 = Wait (ms)(milliseconds to wait="delay before read (ms)") -> ()  [unwired: 1 out]
          }
        }
        n130 = local read "COMBO COMMAND"() -> (w416:string)
        n131 = Search and Replace String(input string=w416, search string="stuff", replace string="1" ("replace string (\"\")")) -> (result string=w422:string)  [unwired: 5 in, 3 out]
        n132 = case shown="\"True\"" w422 {
          tunnel: [FALSE TRUE] -> w419
          frame "False", Default {
          }
          frame "True" {
          }
        }
        n133 = case shown="True" "read" {
          tunnel: w432 -> [w458 w462]
          tunnel: [w458 w466] -> w435
          tunnel: [w457 w465] -> w434
          tunnel: w430 -> [w457 w464]
          frame False {
          }
          frame True {
            # "Read the number of bytes specified."
            n134 = property class="Instr"(reference=w464, error in=w462) -> (reference out=w463:refnum<visa-resource-name>, error out=w461:errorcluster, "Serial Settings:Number of Bytes at Serial Port"=w460:u32)
            "bytes read" <- w460
            n135 = VISA Read(VISA resource name=w463, byte count=w460, error in (no error)=w461) -> (VISA resource name out=w465:refnum<visa-resource-name>, read buffer=→"read string":string, error out=w466:errorcluster)  [unwired: 1 out]
          }
        }
        n136 = Or(x=w419, y=w418) -> (x .or. y?=w417:bool)
        n137 = Wait Until Next ms Multiple(millisecond multiple=u32 50) -> ()  [unwired: 1 out]
      }
      n138 = while {
        shift-right: [w295] -> w36
        shift-left: w52 -> [w297]
        shift-right: [w294] -> w35
        shift-left: w55 -> [w296]
        tunnel: "Quit" -> [w277]
        stop <- w276 stop-if-true
        # "RELAY LV PS"
        # "Configure Serial port (baud rate,\ndata bits, parity, stop bits and flow control)."
        n139 = Match True/False String(2:"" ("false string"), 3:"OUT_SP_00_" ("format string"), 4:"Combo Box 3") -> (0:w287:bool)  [unwired: 1 out]
        n140 = case shown="True" w287 {
          tunnel: [w301 w304] -> w284
          tunnel: "Combo Box 3" -> [w301 w303]
          frame False {
          }
          frame True {
            n141 = Number To Decimal String(number="voltage or current 2") -> (decimal integer string=w306:string)  [unwired: 1 in]
            n142 = Concatenate Strings(w303, w306, "\r\n" ("string")) -> (w304:string)
          }
        }
        "string from combo 3" <- w284
        n143 = case shown="True" "write 3" {
          tunnel: [w311 w316] -> w293
          tunnel: w296 -> [w310 w315]
          tunnel: w297 -> [w311 w314]
          tunnel: [w310 w313] -> w291
          tunnel: w284 -> [_ w312]
          frame False {
          }
          frame True {
            # "Write bytes to port."
            n144 = VISA Write(VISA resource name=w315, write buffer=w312, error in (no error)=w314) -> (VISA resource name out=w313:refnum<visa-resource-name>, error out=w316:errorcluster)  [unwired: 1 out]
          }
        }
        n145 = stacked-sequence {
          tunnel: w293 -> [w309]
          tunnel: [w309] -> w292
          tunnel: w291 -> [w308]
          tunnel: [w308] -> w290
          frame #0 {
            n146 = Wait (ms)(milliseconds to wait="delay before read (ms) 3") -> ()  [unwired: 1 out]
          }
        }
        n147 = local read "COMBO COMMAND"() -> (w278:string)
        n148 = Search and Replace String(input string=w278, search string="stuff", replace string="1" ("replace string (\"\")")) -> (result string=w282:string)  [unwired: 5 in, 3 out]
        n149 = case shown="\"True\"" w282 {
          tunnel: [FALSE TRUE] -> w279
          frame "False", Default {
          }
          frame "True" {
          }
        }
        n150 = case shown="True" "read 3" {
          tunnel: w292 -> [w318 w322]
          tunnel: [w318 w326] -> w295
          tunnel: [w317 w325] -> w294
          tunnel: w290 -> [w317 w324]
          frame False {
          }
          frame True {
            # "Read the number of bytes specified."
            n151 = property class="Instr"(reference=w324, error in=w322) -> (reference out=w323:refnum<visa-resource-name>, error out=w321:errorcluster, "Serial Settings:Number of Bytes at Serial Port"=w320:u32)
            "bytes read 3" <- w320
            n152 = VISA Read(VISA resource name=w323, byte count=w320, error in (no error)=w321) -> (VISA resource name out=w325:refnum<visa-resource-name>, read buffer=→"read string 3":string, error out=w326:errorcluster)  [unwired: 1 out]
          }
        }
        n153 = Or(x=w279, y=w277) -> (x .or. y?=w276:bool)
        n154 = Wait Until Next ms Multiple(millisecond multiple=u32 50) -> ()  [unwired: 1 out]
      }
      n155 = while {
        shift-right: [w346] -> w34
        shift-left: w56 -> [w348]
        shift-right: [w345] -> w33
        shift-left: w59 -> [w347]
        tunnel: "Quit" -> [w333]
        stop <- w332 stop-if-true
        # "TTi SEH PS LV"
        n156 = Match True/False String(2:"" ("false string"), 3:"OUT_SP_00_" ("format string"), 4:"Combo Box 2") -> (0:w338:bool)  [unwired: 1 out]
        n157 = case shown="True" w338 {
          tunnel: [w352 w355] -> w335
          tunnel: "Combo Box 2" -> [w352 w354]
          frame False {
          }
          frame True {
            n158 = Number To Decimal String(number="voltage or current") -> (decimal integer string=w357:string)  [unwired: 1 in]
            n159 = Concatenate Strings(w354, w357, "\r\n" ("string")) -> (w355:string)
          }
        }
        "string from combo 2" <- w335
        n160 = case shown="True" "write 2" {
          tunnel: [w362 w367] -> w344
          tunnel: w347 -> [w361 w366]
          tunnel: w348 -> [w362 w365]
          tunnel: [w361 w364] -> w342
          tunnel: w335 -> [_ w363]
          frame False {
          }
          frame True {
            n161 = VISA Write(VISA resource name=w366, write buffer=w363, error in (no error)=w365) -> (VISA resource name out=w364:refnum<visa-resource-name>, error out=w367:errorcluster)  [unwired: 1 out]
          }
        }
        n162 = stacked-sequence {
          tunnel: w344 -> [w360]
          tunnel: [w360] -> w343
          tunnel: w342 -> [w359]
          tunnel: [w359] -> w341
          frame #0 {
            n163 = Wait (ms)(milliseconds to wait="delay before read (ms) 2") -> ()  [unwired: 1 out]
          }
        }
        n164 = local read "COMBO COMMAND"() -> (w331:string)
        n165 = Search and Replace String(input string=w331, search string="setLVPS", replace string="1" ("replace string (\"\")")) -> (result string=w330:string)  [unwired: 5 in, 3 out]
        n166 = case shown="\"True\"" w330 {
          tunnel: [FALSE TRUE] -> w327
          frame "False", Default {
          }
          frame "True" {
          }
        }
        n167 = case shown="True" "read 2" {
          tunnel: w343 -> [w369 w373]
          tunnel: [w369 w377] -> w346
          tunnel: [w368 w376] -> w345
          tunnel: w341 -> [w368 w375]
          frame False {
          }
          frame True {
            # "Read the number of bytes specified."
            n168 = property class="Instr"(reference=w375, error in=w373) -> (reference out=w374:refnum<visa-resource-name>, error out=w372:errorcluster, "Serial Settings:Number of Bytes at Serial Port"=w371:u32)
            "bytes read 2" <- w371
            n169 = VISA Read(VISA resource name=w374, byte count=w371, error in (no error)=w372) -> (VISA resource name out=w376:refnum<visa-resource-name>, read buffer=→"read string 2":string, error out=w377:errorcluster)  [unwired: 1 out]
          }
        }
        n170 = Or(x=w327, y=w333) -> (x .or. y?=w332:bool)
        n171 = Wait Until Next ms Multiple(millisecond multiple=u32 50) -> ()  [unwired: 1 out]
      }
      n172 = call "Configure Output.vi"("Enable Output (T: Enable)"=w46, "error in (no error)"=w44, "VISA resource name"=w45) -> ("error out"=w48:errorcluster, "VISA resource name out"=w47:refnum<visa-resource-name>)  [unwired: 7 in]
      n173 = while {
        tunnel: "Quit" -> [w66]
        stop <- w65 stop-if-true
        w82 = u16 0 items=["Volts", "Current", "Resistance"]  # Function (0: Volts)
        w89 = u16 2 items=["Volts", "Current", "Resistance"]  # Function (0: Volts)
        w90 = u16 1 items=["Volts", "Current", "Resistance"]  # Function (0: Volts)
        # "Take the readings."
        # "Configure the output."
        # "Configure each of the three measurements. settings"
        n174 = call "Configure Measurement.vi"("Manual Range (1.0)"="Voltage Manual Range (1.0) 2", "Enable Auto Range (T:Enable)"="Enable Voltage Auto Range (T:Enable) 2", "Function (0: Volts)"=w82, "VISA resource name"=refnum<visa-resource-name> "COM1") -> ("error out"=w93:errorcluster, "VISA resource name out"=w94:refnum<visa-resource-name>)  [unwired: 6 in]
        n175 = call "Configure Measurement.vi"("Manual Range (1.0)"="Current Manual Range (1.0) 2", "error in (no error)"=w93, "Enable Auto Range (T:Enable)"="Enable Current Auto Range (T:Enable) 2", "Function (0: Volts)"=w90, "VISA resource name"=w94) -> ("error out"=w92:errorcluster, "VISA resource name out"=w91:refnum<visa-resource-name>)  [unwired: 5 in]
        n176 = call "Configure Measurement.vi"("Manual Range (1.0)"="Resistance Manual Range (1.0) 2", "error in (no error)"=w92, "Enable Auto Range (T:Enable)"="Enable Resistance Auto Range (T:Enable) 2", "Function (0: Volts)"=w89, "VISA resource name"=w91) -> ("error out"=w71:errorcluster, "VISA resource name out"=w72:refnum<visa-resource-name>)  [unwired: 5 in]
        n177 = local read "COMBO COMMAND"() -> (w70:string)
        n178 = call "Enable Output.vi"("error in (no error)"=w71, "Enable Output (T: Enable)"=TRUE, "VISA resource name"=w72) -> ("error out"=w75:errorcluster, "VISA resource name out"=w74:refnum<visa-resource-name>)  [unwired: 7 in]
        n179 = call-poly "Read.vi"("VISA resource name"=w74, "error in (no error)"=w75) -> ("Voltage"=→"Voltage 3":sgl, "Current"=w80:sgl, "Resistance"=→"Resistance 2":sgl)  [unwired: 7 in, 4 out]
        "Current 3" <- w80
        n180 = Search and Replace String(input string=w70, search string="keithleynew", replace string="1" ("replace string (\"\")")) -> (result string=w67:string)  [unwired: 5 in, 3 out]
        n181 = Multiply(x=w80, y=sgl 1000000.0) -> (x*y=→"Current Micro\n 2":sgl)
        n182 = case shown="\"False\", Default" w67 {
          tunnel: [FALSE TRUE] -> w64
          frame "False", Default {
            n183 = Wait (ms)(milliseconds to wait=u32 4000) -> ()  [unwired: 1 out]
          }
          frame "True" {
            n184 = Wait (ms)(milliseconds to wait=u32 4000) -> ()  [unwired: 1 out]
          }
        }
        n185 = Or(x=w66, y=w64) -> (x .or. y?=w65:bool)
      }
      n186 = call "Close.vi"("error in (no error)"=w48, "VISA resource name"=w47) -> ("error out"=w49:errorcluster)  [unwired: 9 in]
      n187 = call <vilib>:"Simple Error Handler.vi"("error in (no error)"=w49) -> ()  [unwired: 4 in, 5 out]
    }
    frame #2 {
      # "Closing things down"
      n188 = VISA Close(VISA resource name=w467, error in (no error)=w468) -> (error out=w469:errorcluster)
      "LV TTi" <- w469
      n189 = call <vilib>:"Simple Error Handler.vi"("error in (no error)"=w469) -> ()  [unwired: 4 in, 5 out]
      n190 = VISA Close(VISA resource name=w470, error in (no error)=w471) -> (error out=w472:errorcluster)
      "relay TTi" <- w472
      n191 = VISA Close(VISA resource name=w473, error in (no error)=w474) -> (error out=w475:errorcluster)
      "Chiller" <- w475
      n192 = call <vilib>:"Simple Error Handler.vi"("error in (no error)"=w472) -> ()  [unwired: 4 in, 5 out]
      n193 = call <vilib>:"Simple Error Handler.vi"("error in (no error)"=w475) -> ()  [unwired: 4 in, 5 out]
      n194 = call "Enable Output.vi"("Enable Output (T: Enable)"=FALSE, "VISA resource name"=refnum<visa-resource-name> "COM1") -> ("error out"=w477:errorcluster, "VISA resource name out"=w478:refnum<visa-resource-name>)  [unwired: 8 in]
      n195 = call "Close.vi"("error in (no error)"=w477, "VISA resource name"=w478) -> ("error out"=w480:errorcluster)  [unwired: 9 in]
      n196 = call <vilib>:"Simple Error Handler.vi"("error in (no error)"=w480) -> ()  [unwired: 4 in, 5 out]
    }
  }
